vi "Custom REST GET.vi"(11 "Base URL":string) -> (0 "Error out":errorcluster, 3 "body":string)   [LabVIEW 2026]
uses:
  <vilib>/httpClient/LabVIEWHTTPClient.lvlib
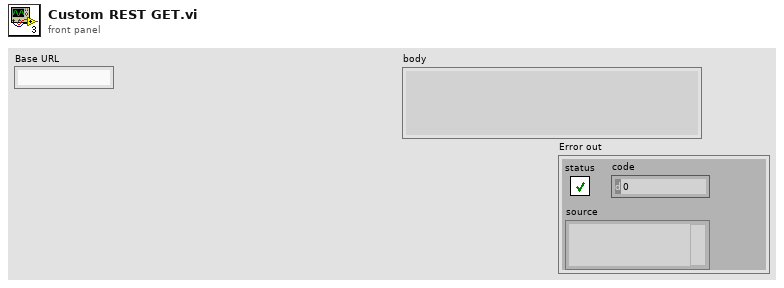
[diagram p1: front panel]
types:
  T1 = typedef "LabVIEWHTTPClient.lvlib/ClientHandle.ctl" = refnum<k1>
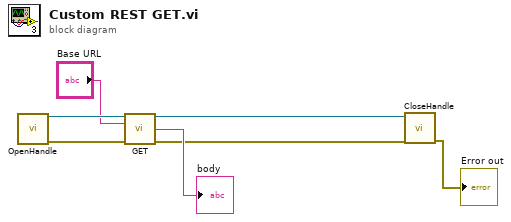
[diagram p0: block diagram]
diagram:
  n1 = call <vilib>:"OpenHandle.vi"() -> ("client handle out"=w7:T1, "error out"=w6:errorcluster)  [unwired: 14 in]
  n2 = call <vilib>:"GET.vi"("client handle"=w7, "url"="Base URL", "error in (no error)"=w6) -> ("client handle out"=w5:T1, "body"=→"body":string, "error out"=w2:errorcluster)  [unwired: 9 in, 1 out]
  n3 = call <vilib>:"CloseHandle.vi"("client handle"=w5, "error in (no error)"=w2) -> ("error out"=→"Error out":errorcluster)  [unwired: 13 in]
